vi "Pop.vi"(11 "ActionStack in":refnum<class "Action.lvclass">[](array[class])) -> (1 "Popped Payload":variant, 2 "Popped Action":string, 3 "Future ActionStack":refnum<class "Action.lvclass">[](array[class]))   [LabVIEW 2025]
uses:
  Action.lvclass
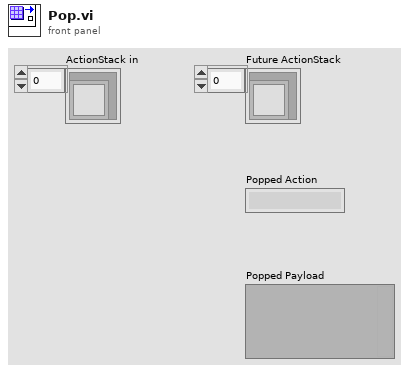
[diagram p1: front panel]
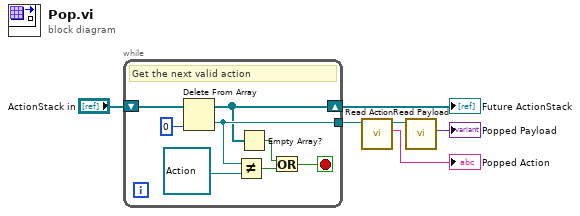
[diagram p0: block diagram]
diagram:
  n1 = while {
    tunnel: [w11] -> w2
    shift-right: [w10] -> w1
    shift-left: "ActionStack in" -> [w14]
    stop <- w7 stop-if-true
    # "Get the next valid action"
    n2 = Delete From Array(array=w14, index=0) -> (deleted portion=w11:refnum<class "Action.lvclass">, array with subset deleted=w10:refnum<class "Action.lvclass">[])  [unwired: 1 in]
    n3 = Not Equal?(x=w11, y=refnum<class "Action.lvclass"> refnum ("ActionStack out")) -> (x != y?=w8:bool)
    n4 = Empty Array?(array=w10) -> (empty?=w9:bool)
    n5 = Or(x=w9, y=w8) -> (x .or. y?=w7:bool)
  }
  "Future ActionStack" <- w1
  n6 = call-dynamic "Read Action.vi"("ActionStack in"=w2) -> ("Action"=→"Popped Action":string, "ActionStack out"=w5:refnum<class "Action.lvclass">)  [unwired: 9 in]
  n7 = call-dynamic "Read Payload.vi"("ActionStack in"=w5) -> ("Payload"=→"Popped Payload":variant)  [unwired: 9 in, 1 out]
